vi "ParseData1.vi"(4 "data out":string) -> (0 "senso id(b)":u8, 1 "Sensor data(b)":T1, 2 "senso id":u8, 5 "Sensor data (a)":T1)   [LabVIEW 2011]
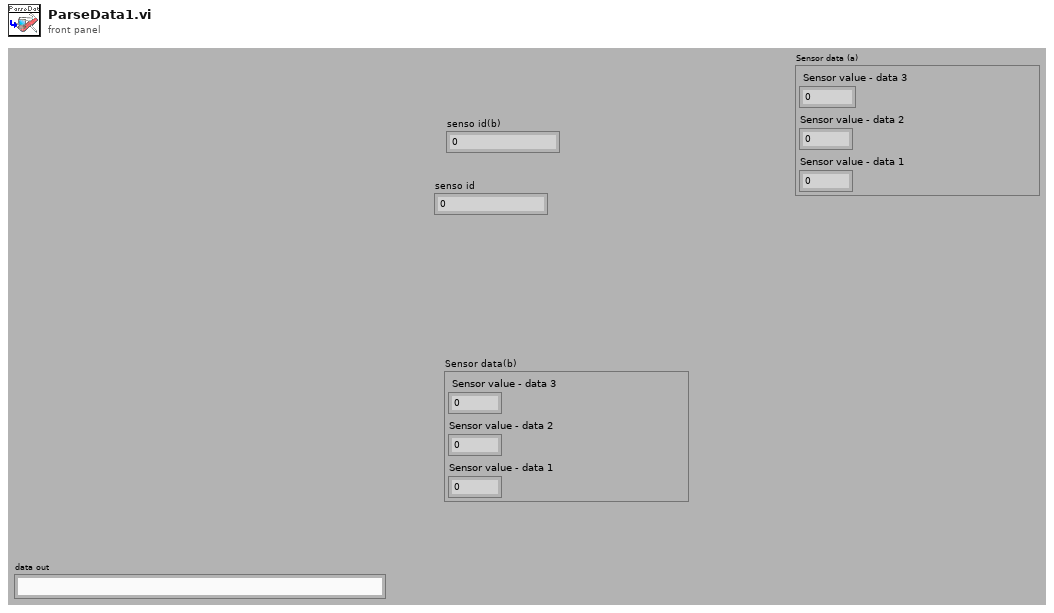
[diagram p1: front panel]
types:
  T1 = cluster{" Sensor value - data 3":u16, "Sensor value - data 2":u16, "Sensor value - data 1":u16}
  T2 = cluster{"sp float":u16, "sp float":u16, "index":i32}
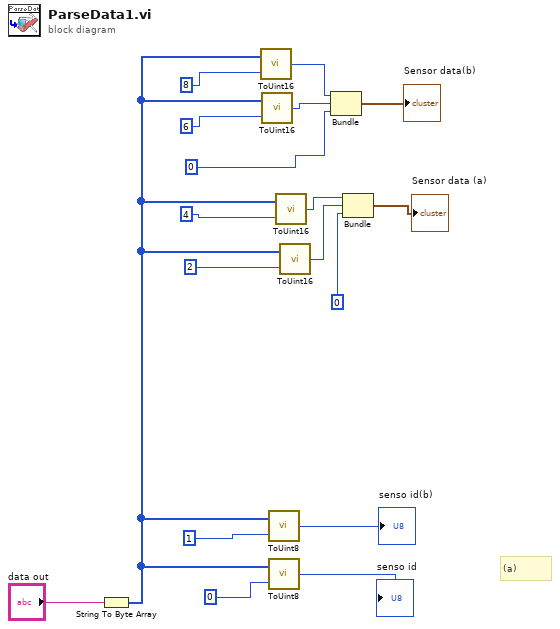
[diagram p0: block diagram]
diagram:
  # "(a)"
  n1 = String To Byte Array(string="data out") -> (unsigned byte array=w2:u8[])
  n2 = call "ToUint16.vi"("index"=8, "array"=w2) -> ("sp float"=w15:u16)
  n3 = call "ToUint16.vi"("index"=6, "array"=w2) -> ("sp float"=w14:u16)
  n4 = call "ToUint8.vi"("index"=1, "array"=w2) -> ("sp float"=→"senso id(b)":u8)
  n5 = call "ToUint8.vi"("index"=0, "array"=w2) -> ("sp float"=→"senso id":u8)
  n6 = call "ToUint16.vi"("index"=4, "array"=w2) -> ("sp float"=w6:u16)
  n7 = call "ToUint16.vi"("index"=2, "array"=w2) -> ("sp float"=w5:u16)
  n8 = Bundle("sp float"=w15, "sp float"=w14, "index"=0) -> (→"Sensor data(b)":T2)  [unwired: 1 in]
  n9 = Bundle("sp float"=w6, "sp float"=w5, "index"=0) -> (→"Sensor data (a)":T2)  [unwired: 1 in]
